vi "ex1.vi"() -> ()   [LabVIEW 2017]
uses:
  <vilib>/sound2/lvsound2.llb/Sound Data Format.ctl
  <vilib>/sound2/lvsound2.llb/Sampling Mode.ctl
  <vilib>/sound2/lvsound2.llb/Sound Input Read (DBL).vi
  <vilib>/measure/maspectr.llb/FFT Power Spectrum and PSD for N Chan.vi
  <vilib>/addons/_NISVFA/_Subset FFT/SVFA Power Spectrum Subset (N Ch).vi
  <vilib>/measure/NI_MAPro.lvlib
panel:
  out "FFT Power Spectrum":cluster{"f0":dbl, "df":dbl, "magnitude":dbl[]}[](graph)
  out "Time Signal":waveform(dbl)[](graph)
  out "SVFA Power Spectrum":cluster{"f0":dbl, "df":dbl, "magnitude":dbl[]}[](graph)
  in  "stop":bool
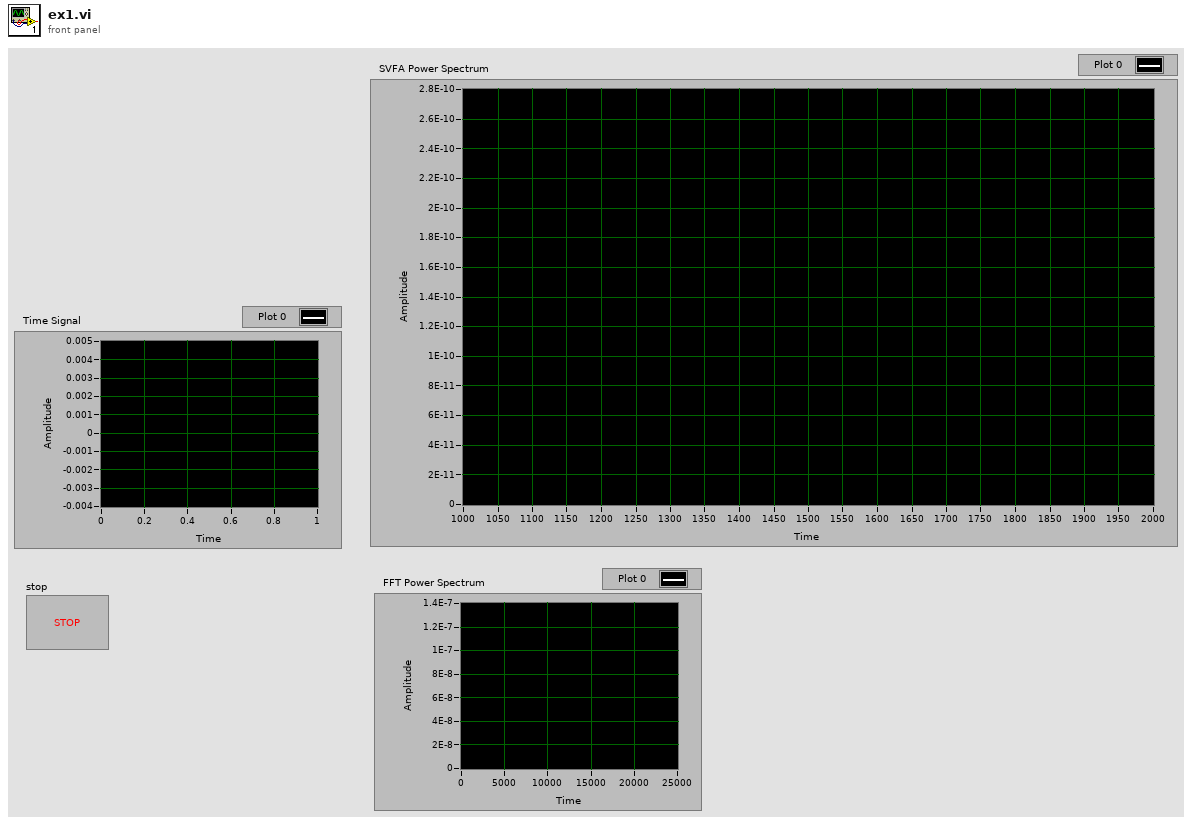
[diagram p1: front panel]
types:
  T1 = typedef "Sampling Mode.ctl" = i32
  T2 = typedef "Sound Data Format.ctl" = cluster{"sample rate (S/s)":dbl, "number of channels":i32, "bits per sample":i32}
  T3 = typedef "Sound Input Task ID.ctl" = u32
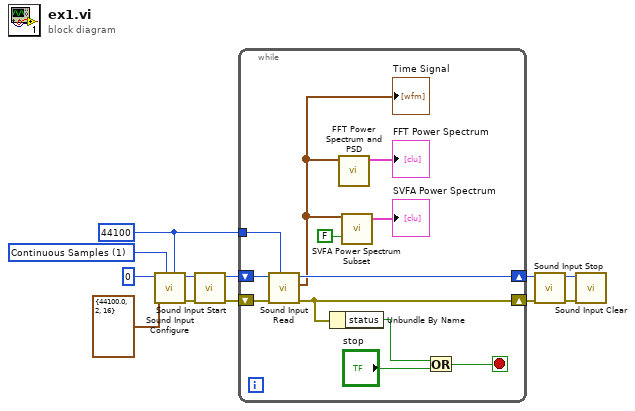
[diagram p0: block diagram]
diagram:
  w1 = 44100 ("number of samples/ch")
  w6 = T1 1 items=["Finite Samples", "Continuous Samples"] ("sample mode")
  n1 = call <vilib>:"Sound Input Configure.vi"("number of samples/ch"=w1, "sample mode"=w6, "sound format"=T2 {"sample rate (S/s)"=44100.0, "number of channels"=2, "bits per sample"=16}, "device ID"=u32 0) -> ("error out"=w10:errorcluster, "task ID"=w5:T3)  [unwired: 6 in]
  n2 = call <vilib>:"Sound Input Start.vi"("error in (no error)"=w10, "task ID"=w5) -> ("error out"=w9:errorcluster, "task ID out"=w4:T3)  [unwired: 8 in]
  n3 = while {
    shift-right: [w21] -> w8
    shift-left: w9 -> [w24]
    shift-right: [w22] -> w2
    shift-left: w4 -> [w23]
    tunnel: w1 -> [w14]
    stop <- w18 stop-if-true
    n4 = call-poly <vilib>:"Sound Input Read.vi"("number of samples/ch"=w14, "error in (no error)"=w24, "task ID"=w23) -> ("error out"=w21:errorcluster, "data"=w15:waveform(dbl)[], "task ID out"=w22:T3)  [unwired: 6 in]
    "Time Signal" <- w15
    n5 = Unbundle By Name(w21) -> ("status"=w20:bool)
    n6 = call-poly <vilib>:"FFT Power Spectrum and PSD.vi"("time signals"=w15) -> ("Power Spectrum / PSD"=→"FFT Power Spectrum":cluster{"f0":dbl, "df":dbl, "magnitude":dbl[]}[])  [unwired: 7 in, 3 out]
    n7 = call-poly <vilib>:"SVFA Power Spectrum Subset.vi"("scaled signals [EU]"=w15, "dB On (T)"=FALSE) -> ("power spectra [dB EU]"=→"SVFA Power Spectrum":cluster{"f0":dbl, "df":dbl, "magnitude":dbl[]}[])  [unwired: 12 in, 5 out]
    n8 = Or(x=w20, y="stop") -> (x .or. y?=w18:bool)
  }
  n9 = call <vilib>:"Sound Input Stop.vi"("error in (no error)"=w8, "task ID"=w2) -> ("error out"=w7:errorcluster, "task ID out"=w3:T3)  [unwired: 8 in]
  n10 = call <vilib>:"Sound Input Clear.vi"("error in (no error)"=w7, "task ID"=w3) -> ()  [unwired: 9 in, 1 out]
